vi "FTW-ActorConfig-FormatExtendedSubscriptions.vi"(0 "FTW Config String In":string="{}", 5 "Subscription Names":string[](array[string]), 7 "Subscription Addresses":string[](array[string]), 9 "Subscriber Depth":i32=1, 11 "error in":errorcluster) -> (4 "FTW Config String":string, 15 "error out":errorcluster)   [LabVIEW 2015]
uses:
  container/FTW-Container.lvclass
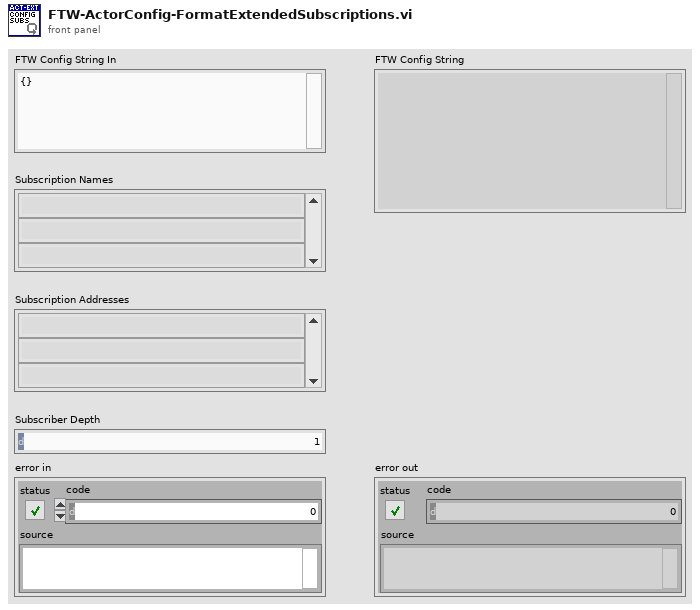
[diagram p1: front panel]
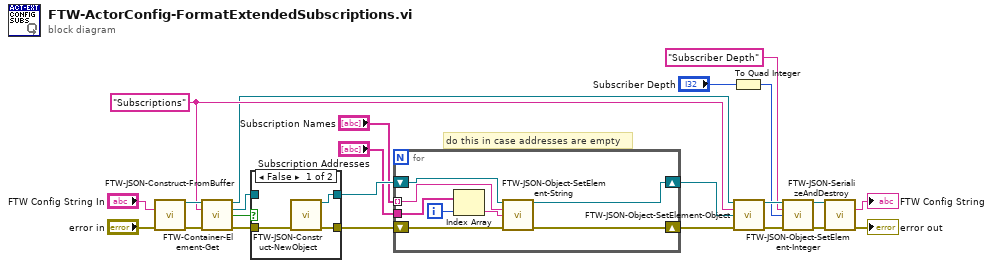
[diagram p0: block diagram]
diagram:
  w11 = "Subscriptions" ("Element Name")
  # "do this in case addresses are empty"
  n1 = call "FTW-JSON-Construct-FromBuffer.vi"("JSON String (UTF-8)"="FTW Config String In", "error in"="error in") -> ("JSON"=w22:refnum<class "FTW-Container.lvclass">, "error out"=w21:errorcluster)  [unwired: 12 in]
  n2 = call "FTW-Container-Element-Get.vi"("FTW-Container In"=w22, "Element Name"=w11, "error in"=w21) -> ("FTW-Container Out"=w10:refnum<class "FTW-Container.lvclass">, "Element Out"=w19:refnum<class "FTW-Container.lvclass">, "Found"=w20:bool, "error out"=w18:errorcluster)  [unwired: 9 in]
  n3 = case shown="False" w20 {
    tunnel: w19 -> [_ w29]
    tunnel: w18 -> [w27 w28]
    tunnel: [w26 w29] -> w16
    tunnel: [w25 w28] -> w17
    frame False {
      n4 = call "FTW-JSON-Construct-NewObject.vi"("error in"=w27) -> ("JSON"=w26:refnum<class "FTW-Container.lvclass">, "error out"=w25:errorcluster)  [unwired: 13 in]
    }
    frame True {
    }
  }
  n5 = for {
    tunnel: "Subscription Names" -> [w35] mode=indexing
    shift-right: [w34] -> w14
    shift-left: w17 -> [w37]
    shift-right: [w33] -> w13
    shift-left: w16 -> [w36]
    tunnel: "Subscription Addresses" -> [w32]
    i -> [w30]
    n6 = Index Array(array=w32, index=w30) -> (element=w31:string)
    n7 = call "FTW-JSON-Object-SetElement-String.vi"("JSON"=w36, "Key"=w35, "Value"=w31, "error in"=w37) -> ("JSON out"=w33:refnum<class "FTW-Container.lvclass">, "error out"=w34:errorcluster)  [unwired: 10 in]
  }
  n8 = To Quad Integer(1:"Subscriber Depth") -> (0:w2:i64)
  n9 = call "FTW-JSON-Object-SetElement-Object.vi"("JSON Object"=w10, "Key"=w11, "JSON Sub-Object"=w13, "error in"=w14) -> ("JSON Root Object"=w5:refnum<class "FTW-Container.lvclass">, "error out"=w9:errorcluster)  [unwired: 10 in]
  n10 = call "FTW-JSON-Object-SetElement-Integer.vi"("JSON"=w5, "Key"="Subscriber Depth", "Value"=w2, "error in"=w9) -> ("JSON out"=w4:refnum<class "FTW-Container.lvclass">, "error out"=w6:errorcluster)  [unwired: 10 in]
  n11 = call "FTW-JSON-SerializeAndDestroy.vi"("JSON"=w4, "error in"=w6) -> ("JSON String (UTF-8)"=→"FTW Config String":string, "error out"=→"error out":errorcluster)  [unwired: 12 in]
